vi "DSF.Shared.Configuration.Framework.Set Transfer Group Configurations.vi"(10 "Transfer Group Configurations":refnum<class "DSF.Shared.Configuration.Transfer Group.lvclass">[](array[class]), 11 "Framework Configuration in":refnum<class "DSF.Shared.Configuration.Framework.lvclass">) -> (3 "Framework Configuration out":refnum<class "DSF.Shared.Configuration.Framework.lvclass">)   [LabVIEW 2017, in "DSF.Shared.lvlib" / "DSF.Shared.Configuration.Framework.lvclass"]
uses:
  DSF.Shared.Configuration.Framework.lvclass
  Transfer Group/DSF.Shared.Configuration.Transfer Group.lvclass
  DSF.Shared.Configuration.Framework.lvclass/DSF.Shared.Configuration.Framework.ctl
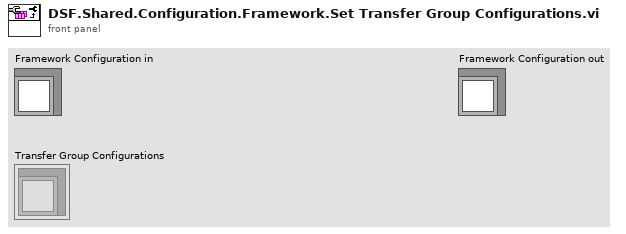
[diagram p1: front panel]
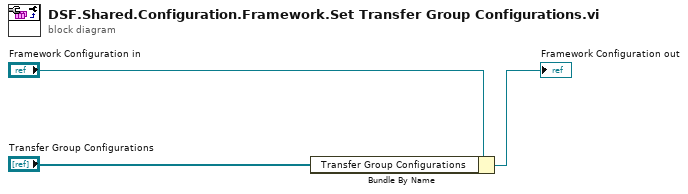
[diagram p0: block diagram]
diagram:
  n1 = Bundle By Name(cluster="Framework Configuration in", "Transfer Group Configurations"="Transfer Group Configurations") -> (→"Framework Configuration out":refnum<class "DSF.Shared.Configuration.Framework.lvclass">)
